vi "read.vi"(8 "error in (no error)":errorcluster, 10 "block size":i32, 11 "SignalReader in":refnum<class "SignalReaderCN091129DAQmx.lvclass">) -> (0 "error out":errorcluster, 1 "finished?":bool, 2 "signals read":dbl[][](graph), 3 "SignalReader out":refnum<class "SignalReaderCN091129DAQmx.lvclass">, 4 "buffer overflow?":bool)   [LabVIEW 2010, in "SignalReaderCN091129DAQmx.lvclass"]
uses:
  SignalReaderCN091129DAQmx.lvclass
  SignalReaderCN091129DAQmx.lvclass/SignalReaderCN091129DAQmx.ctl
  GenericSignalReader/GenericSignalReader/GenericSignalReader.lvclass
  <vilib>/DAQmx/read.llb/DAQmx Read (Analog 2D DBL NChan NSamp).vi
  <vilib>/daqmx/miscellaneous.llb/DAQmx Fill In Error Info.vi
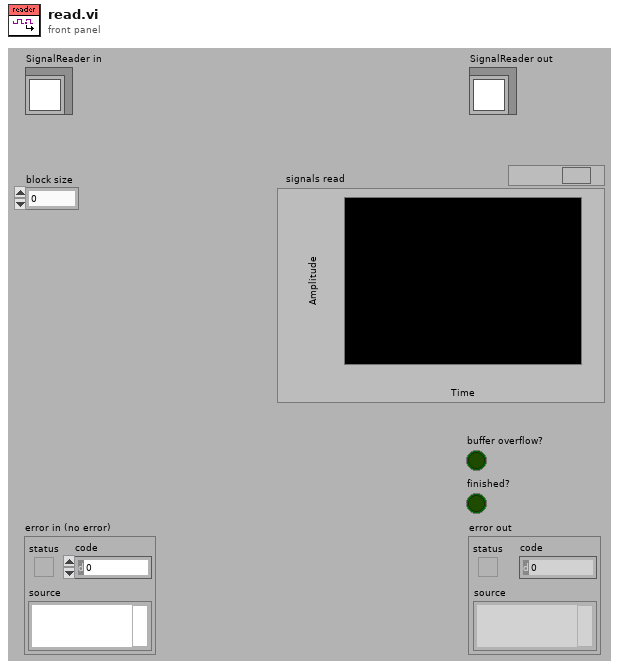
[diagram p1: front panel]
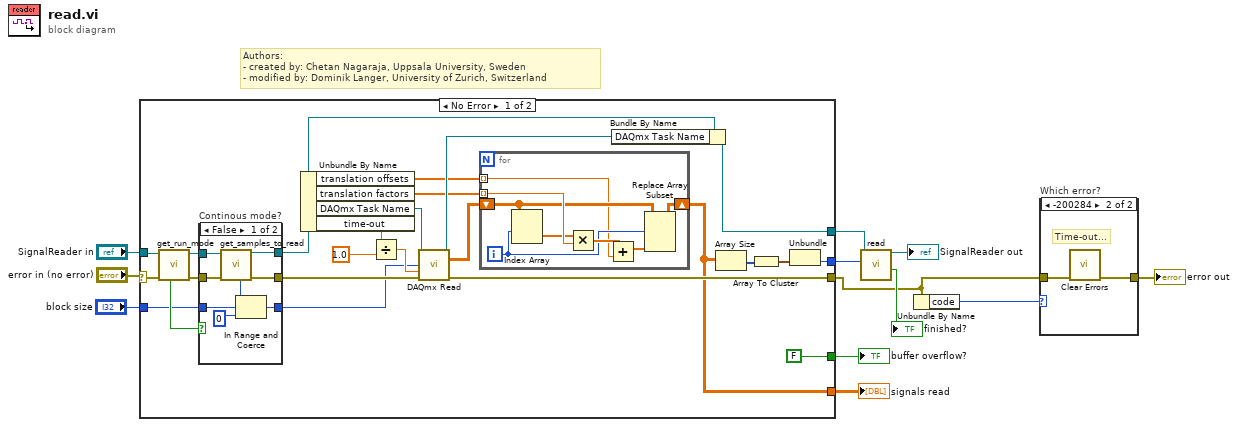
[diagram p0: block diagram]
diagram:
  # "Authors: \n- created by: Chetan Nagaraja, Uppsala University, Sweden\n- modified by: Dominik Langer, University of Zurich, Switzerland"
  n1 = case shown="No Error" "error in (no error)" {
    selector: "error in (no error)" -> [w28 w57]
    tunnel: [w16 w57] -> w1
    tunnel: "SignalReader in" -> [w26 w56]
    tunnel: [w36 w56] -> w9
    tunnel: [w14 _] -> w6
    tunnel: [FALSE _] -> w10
    tunnel: "block size" -> [w22 _]
    tunnel: [w19 _] -> w5
    frame No Error {
      n2 = call-dynamic "get_run_mode.vi"("error in (no error)"=w28, "GenericPlugin in"=w26) -> ("error out"=w27:errorcluster, "GenericPlugin out"=w25:refnum<class "SignalReaderCN091129DAQmx.lvclass">, "is free run?"=w24:bool)  [unwired: 5 in, 2 out]
      n3 = case "Continous mode?" shown="False" w24 {
        tunnel: [w52 w53] -> w30
        tunnel: [w50 w54] -> w29
        tunnel: w22 -> [w48 w55]
        tunnel: [w47 w55] -> w23
        tunnel: w27 -> [w46 w53]
        tunnel: w25 -> [w45 w54]
        frame False {
          n4 = call-dynamic "get_samples_to_read.vi"("error in (no error)"=w46, "GenericSignalReader in"=w45) -> ("error out"=w52:errorcluster, "GenericSignalReader out"=w50:refnum<class "SignalReaderCN091129DAQmx.lvclass">, "samples still to be read"=w49:i32)  [unwired: 5 in, 2 out]
          n5 = In Range and Coerce(upper limit=w49, x=w48, lower limit=0) -> (coerced(x)=w47:i32)  [unwired: 1 out]
        }
        frame True {
        }
      }
      n6 = Unbundle By Name(w29) -> ("translation offsets"=w13:dbl[], "translation factors"=w18:dbl[], "DAQmx Task Name"=w15:refnum<k21>, "time-out"=w33:dbl[unit])
      n7 = Divide(x=w33, y=dbl[unit] 1.0) -> (x/y=w31:dbl)
      n8 = call-poly <vilib>:"DAQmx Read.vi"("task/channels in"=w15, "number of samples per channel"=w23, "timeout"=w31, "error in"=w30) -> ("task out"=w35:refnum<k21>, "data"=w17:dbl[][], "error out"=w16:errorcluster)  [unwired: 9 in]
      n9 = for {
        tunnel: w18 -> [w44] mode=indexing
        shift-right: [w42] -> w14
        shift-left: w17 -> [w43]
        tunnel: w13 -> [w37] mode=indexing
        i -> [w39]
        n10 = Index Array(array=w43, index (row)=w39) -> (element=w41:dbl[])  [unwired: 1 in]
        n11 = Multiply(x=w44, y=w41) -> (x*y=w40:dbl[])
        n12 = Add(x=w40, y=w37) -> (x+y=w38:dbl[])
        n13 = Replace Array Subset(array=w43, new element=w38, index (row)=w39) -> (w42:dbl[][])  [unwired: 1 in]
      }
      n14 = Bundle By Name(cluster=w29, "DAQmx Task Name"=w35) -> (w36:refnum<class "SignalReaderCN091129DAQmx.lvclass">)
      n15 = Array Size(array=w14) -> (size(s)=w21:i32[])
      n16 = Array To Cluster(array=w21) -> (cluster=w20:cluster{"[0]":i32, "[1]":i32})
      n17 = Unbundle(w20) -> ("[1]"=w19:i32)  [unwired: 1 out]
    }
    frame Error {
    }
  }
  "buffer overflow?" <- w10
  "signals read" <- w6
  n18 = call-parent "read.vi"("block size"=w5, "SignalReader in"=w9) -> ("finished?"=→"finished?":bool, "SignalReader out"=→"SignalReader out":refnum<class "SignalReaderCN091129DAQmx.lvclass">)  [unwired: 5 in, 3 out]
  n19 = Unbundle By Name(w1) -> ("code"=w4:i32)
  n20 = case "Which error?" shown="-200284" w4 {
    tunnel: w1 -> [w58 w60]
    tunnel: [w58 w59] -> w3
    frame 0, Default {
    }
    frame -200284 {
      # "Time-out..."
      n21 = call <vilib>:"Clear Errors.vi"("error in (no error)"=w60) -> ("error out"=w59:errorcluster)  [unwired: 6 in]
    }
  }
  "error out" <- w3
